vi "Stop Core.vi"(10 "final error code":i32, 11 "Door Hardware in":refnum<class "Door Hardware.lvclass">) -> (3 "Door Hardware out":refnum<class "Door Hardware.lvclass">)   [LabVIEW 2020, in "Door Hardware.lvlib" / "Door Hardware.lvclass"]
doc: "(<B>Filename</B>: Actor Framework.lvlib:Actor.lvclass:Stop Core.vi)\n\nDefines what the actor does before it stops. Use the <B>final error code</B> input to determine whether the actor shut down in response to an error.\n\nBy default, this method passes the Stop message along to all auto-stop nested actors. A descendant class may override this method to define additional behavior, such as shutting down any processes the actor initiated in its override of the Actor Core method."
uses:
  Door Hardware.lvclass
  <vilib>/ActorFramework/Time-Delayed Send Message/Time-Delay Override Options.ctl
  Door Hardware.lvclass/Door Hardware.ctl
  Application/Application/Application.lvclass
  Door Interlocks/Door Interlocks.lvclass
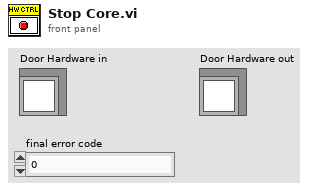
[diagram p1: front panel]
types:
  T1 = typedef "Time-Delay Override Options.ctl" = enum16{"Send next copy now", "Skip next scheduled copy", "Send next copy now and stop all further copies", "Stop all further copies"}
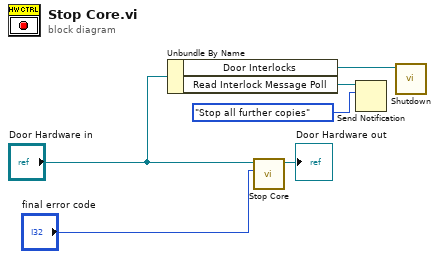
[diagram p0: block diagram]
diagram:
  n1 = Unbundle By Name("Door Hardware in") -> ("Door Interlocks"=w1:refnum<class "Door Interlocks.lvclass">, "Read Interlock Message Poll"=w2:refnum<notifier>)
  n2 = call-parent "Stop Core.vi"("final error code"="final error code", "Actor in"="Door Hardware in") -> ("Actor out"=→"Door Hardware out":refnum<class "Door Hardware.lvclass">)  [unwired: 9 in]
  n3 = Send Notification(notification=Time-Delay_Override_Options."Stop all further copies", notifier=w2) -> ()  [unwired: 1 in, 2 out]
  n4 = call-dynamic "Shutdown.vi"("Door Interlocks in"=w1) -> ()  [unwired: 9 in, 2 out]
